vi "Simple_DAQ_AnalogIO.destroy DAQ channels.vi"(0 "i ref in":refnum<vi>, 3 "Timeout":i32=10000, 5 "error in":errorcluster caption="Fehler (Eingang, kein Fehler)") -> (14 "i ref out":refnum<vi>, 19 "error out":errorcluster caption="Fehler (Ausgang)")   [LabVIEW 2014, in "Simple_DAQ_AnalogIO.lvlib"]
doc: "Contact: Falk Ziegler, info@lab-coding.de"
uses:
  Simple_DAQ_AnalogIO.lvlib
  <vilib>/DAQmx/write.llb/DAQmx Write (Analog DBL 1Chan 1Samp).vi
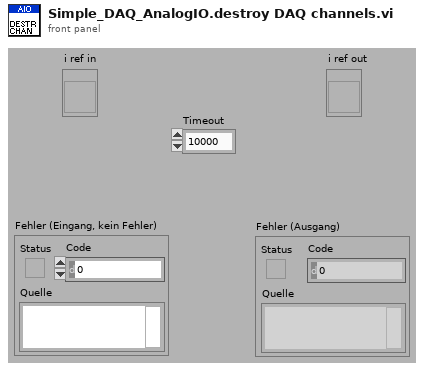
[diagram p1: front panel]
types:
  T1 = typedef "Simple_DAQ_AnalogIO.lvlib/Simple_DAQ_AnalogIO.i attribute.ctl" = cluster{"inputs":cluster{"index":i32[], "channel_task":refnum<k21>[], "range":cluster{"min":dbl, "max":dbl}[], "channel_number":i32, "scale_factor":dbl}, "outputs":cluster{"index":i32[], "channel_task":refnum<k21>[], "range":cluster{"min":dbl, "max":dbl}[], "channel_number":i32, "scale_factor":dbl}}
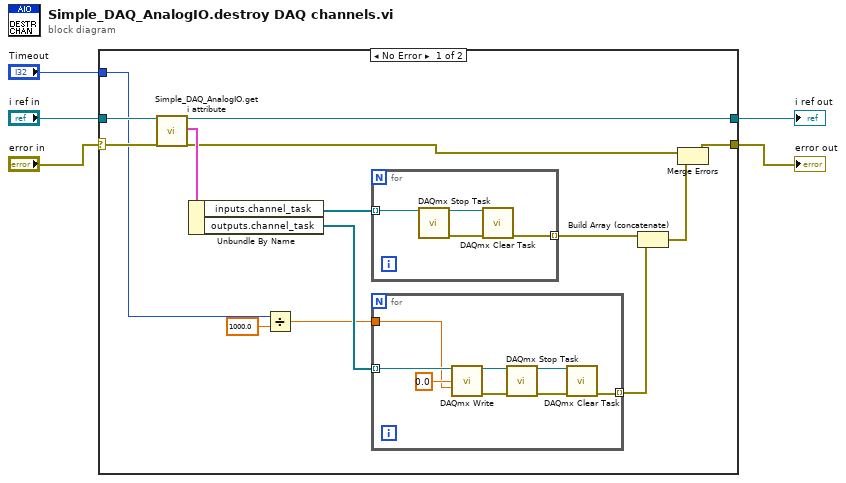
[diagram p0: block diagram]
diagram:
  n1 = case shown="No Error" "error in" {
    selector: "error in" -> [w18 w33]
    tunnel: "i ref in" -> [w19 w32]
    tunnel: [w9 w33] -> w3
    tunnel: [w17 w32] -> w2
    tunnel: "Timeout" -> [w7 _]
    frame No Error {
      n2 = call "Simple_DAQ_AnalogIO.get i attribute.vi"("i ref in"=w19, "error in (no error)"=w18) -> ("i ref out"=w17:refnum<vi>, "i attribute"=w16:T1, "error out"=w13:errorcluster)  [unwired: 15 in]
      n3 = Unbundle By Name(w16) -> ("inputs.channel_task"=w15:refnum<k21>[], "outputs.channel_task"=w14:refnum<k21>[])
      n4 = Divide(x=w7, y=1000.0) -> (x/y=w6:dbl)
      n5 = for {
        tunnel: w15 -> [w23] mode=indexing
        tunnel: [w20] -> w12 mode=indexing
        n6 = call <vilib>:"DAQmx Stop Task.vi"("task/channels in"=w23) -> ("task out"=w22:refnum<k21>, "error out"=w21:errorcluster)  [unwired: 13 in]
        n7 = call <vilib>:"DAQmx Clear Task.vi"("task in"=w22, "error in"=w21) -> ("error out"=w20:errorcluster)  [unwired: 13 in]
      }
      n8 = for {
        tunnel: w14 -> [w31] mode=indexing
        tunnel: [w25] -> w11 mode=indexing
        tunnel: w6 -> [w24]
        n9 = call-poly <vilib>:"DAQmx Write.vi"("task/channels in"=w31, "data"=0.0, "timeout"=w24) -> ("task out"=w29:refnum<k21>, "error out"=w27:errorcluster)  [unwired: 10 in, 1 out]
        n10 = call <vilib>:"DAQmx Stop Task.vi"("task/channels in"=w29, "error in"=w27) -> ("task out"=w28:refnum<k21>, "error out"=w26:errorcluster)  [unwired: 12 in]
        n11 = call <vilib>:"DAQmx Clear Task.vi"("task in"=w28, "error in"=w26) -> ("error out"=w25:errorcluster)  [unwired: 13 in]
      }
      n12 = Build Array (concatenate)(w12, w11) -> (w10:errorcluster[])
      n13 = Merge Errors(w13, w10) -> (w9:errorcluster)
    }
    frame Error {
    }
  }
  "error out" <- w3
  "i ref out" <- w2
